vi "MecanumSpeedControlDrive.vi"(0 "RobotDriveDevRef":T1={"DevStatus"={"status"=FALSE, "code"=0, "source"=""}, "Motors[]"=[], "Square Inputs"=FALSE, "Max Output"=1.0}, 1 "Gyro Angle":dbl, 5 "X":dbl, 7 "Array":dbl[](array[numeric]), 9 "Y":dbl, 11 "error in (no error)":errorcluster, 12 "Rotation":dbl) -> (4 "RobotDriveDevRef":T1={"DevStatus"={"status"=FALSE, "code"=0, "source"=""}, "Motors[]"=[], "Square Inputs"=FALSE, "Max Output"=1.0}, 6 "Motor Values":dbl[](array[numeric]), 15 "error out":errorcluster)   [LabVIEW 2014]
doc: "Configures the motors for holonomic driving. Holonomic driving allows you to move the robot in any direction without first rotating or maneuvering the robot.\n\nThis VI requires the robot to have either four omni-directional wheels and four motors mounted at 45 degree angles in the four corners of a square frame or to have four mecanum wheels driven by four motors.\n\nThe control input is intended to be connected directly to the X, Y, and Z axes of a joystick. The Y axis is inverted for you.\n\nThis software is licensed. Open the labview\\readme\\WPI Robotics Library Open Source License.txt file for more information."
uses:
  <vilib>/Rock Robotics/WPI/RobotDrive/WPI_RobotDriveDevRef.ctl
  <vilib>/Rock Robotics/WPI/MotorControl/WPI_MotorControlDeviceRef.ctl
  <vilib>/Rock Robotics/WPI/MotorControl/WPI_MotorControlType.ctl
  <vilib>/Rock Robotics/SystemInterfaces/Typedef/FPGA_TypedefDigitalModule.ctl
  <vilib>/Rock Robotics/SystemInterfaces/DIO/FPGA_DIOPWMChannel.ctl
  <vilib>/Rock Robotics/WPI/PWM/WPI_PWMDeadband.ctl
  <vilib>/Rock Robotics/WPI/CAN/Jaguar/SubVIs/WPI_CANJaguar_ControlMode.ctl
  <vilib>/Rock Robotics/WPI/CAN/TalonSRX/WPI_CANTalonSRX_APIControlMode.ctl
  <vilib>/Rock Robotics/WPI/PWM/WPI_PWMTransform_ConPane.ctl
  <vilib>/Rock Robotics/SystemInterfaces/NetworkCommunication/NetComm_UsageReport_ResourceType.ctl
  <vilib>/Rock Robotics/WPI/RobotDrive/WPI_RobotDriveMotorSelectorEnum.ctl
  <vilib>/Rock Robotics/WPI/RobotDrive/WPI_RobotDriveSafetyCheck.vi
panel:
  out "Front Right":dbl(graph)
  out "Rear Left":dbl(graph)
  out "Rear Right":dbl(graph)
  out "Front Left":dbl(graph)
  out "Right Front":dbl(graph)
  out "Left Front":dbl(graph)
  out "Right Rear":dbl(graph)
  out "Left Rear":dbl(graph)
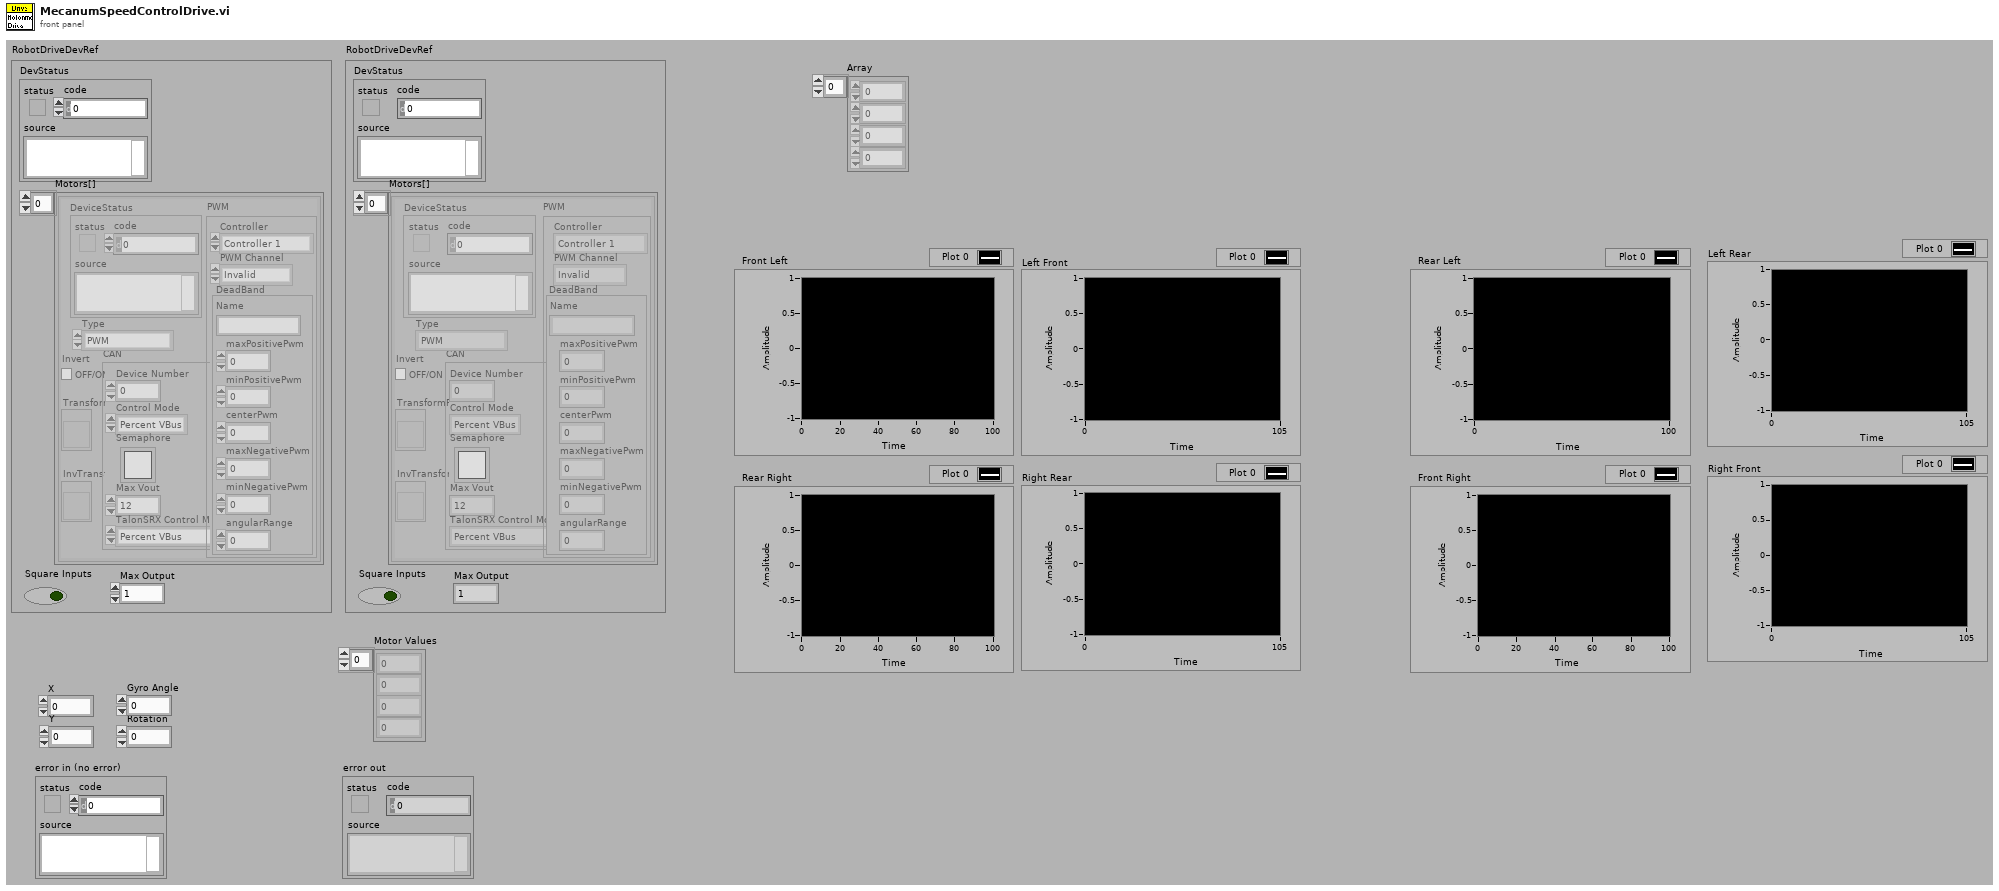
[diagram p1: front panel]
types:
  T1 = typedef "WPI_RobotDriveDevRef.ctl" = cluster{"DevStatus":errorcluster, "Motors[]":T2[], "Square Inputs":bool, "Max Output":dbl}
  T2 = typedef "WPI_MotorControlDeviceRef.ctl" = cluster{"DeviceStatus":errorcluster, "Type":T3, "PWM":cluster{"Controller":T4, "PWM Channel":T5, "DeadBand":T6}, "CAN":cluster{"Device Number":u8, "Control Mode":T7, "Semaphore":T8, "Max Vout":dbl, "TalonSRX Control Mode":T9}, "Invert":bool, "TransformRef":T10, "InvTransformRef":T10}
  T3 = typedef "WPI_MotorControlType.ctl" = enum16{"PWM", "CAN", "CANTalonSRX"}
  T4 = typedef "FPGA_TypedefDigitalModule.ctl" = enum16{"Controller 1"}
  T5 = typedef "FPGA_DIOPWMChannel.ctl" = enum8{"PWM 0", "PWM 1", "PWM 2", "PWM 3", "PWM 4", "PWM 5", "PWM 6", "PWM 7", "PWM 8", "PWM 9", "PWM MXP 0", "PWM MXP 1", "PWM MXP 2", "PWM MXP 3", "PWM MXP 4", "PWM MXP 5", "PWM MXP 6", "PWM MXP 7", "PWM MXP 8", "PWM MXP 9", "Invalid"}
  T6 = typedef "WPI_PWMDeadband.ctl" = cluster{"Name":string, "maxPositivePwm":i32, "minPositivePwm":i32, "centerPwm":i32, "maxNegativePwm":i32, "minNegativePwm":i32, "angularRange":u16}
  T7 = typedef "WPI_CANJaguar_ControlMode.ctl" = enum8{"Percent VBus", "Current", "Speed", "Position", "Voltage"}
  T8 = typedef "Semaphore RefNum" = refnum<k1>
  T9 = typedef "WPI_CANTalonSRX_APIControlMode.ctl" = enum8{"Percent VBus", "Speed", "Position", "Slave", "Unchanged / Invalid"}
  T10 = typedef "WPI_PWMTransform_ConPane.ctl" = refnum<vi>
  T11 = typedef "NetComm_UsageReport_ResourceType.ctl" = enum8{"Controller", "Module", "Language", "CANPlugin", "Accelerometer", "ADXL345", "AnalogChannel", "AnalogTrigger", "AnalogTriggerOutput", "CANJaguar", "Compressor", "Counter", "Dashboard", "DigitalInput", "DigitalOutput", "DriverStationCIO", "DriverStationEIO", "DriverStationLCD", "Encoder", "GearTooth", "Gyro", "I2C", "Framework", "Jaguar", "Joystick", "Kinect", "KinectStick", "PIDController", "Preferences", "PWM", "Relay", "RobotDrive", "SerialPort", "Servo", "Solenoid", "SPI", "Task", "Ultrasonic", "Victor", "Button", "Command", "AxisCamera", "PCVideoServer", "SmartDashboard", "Talon", "HiTechnicColorSensor", "HiTechnicAccel", "HiTechnicCompass", "SRF08", "AnalogOutput", "Victor SP", "Talon SRX", "CAN Talon SRX"}
  T12 = typedef "WPI_RobotDriveMotorSelectorEnum.ctl" = enum16{"Rear Left Motor", "Rear Right Motor", "Front Left Motor", "Front Right Motor"}
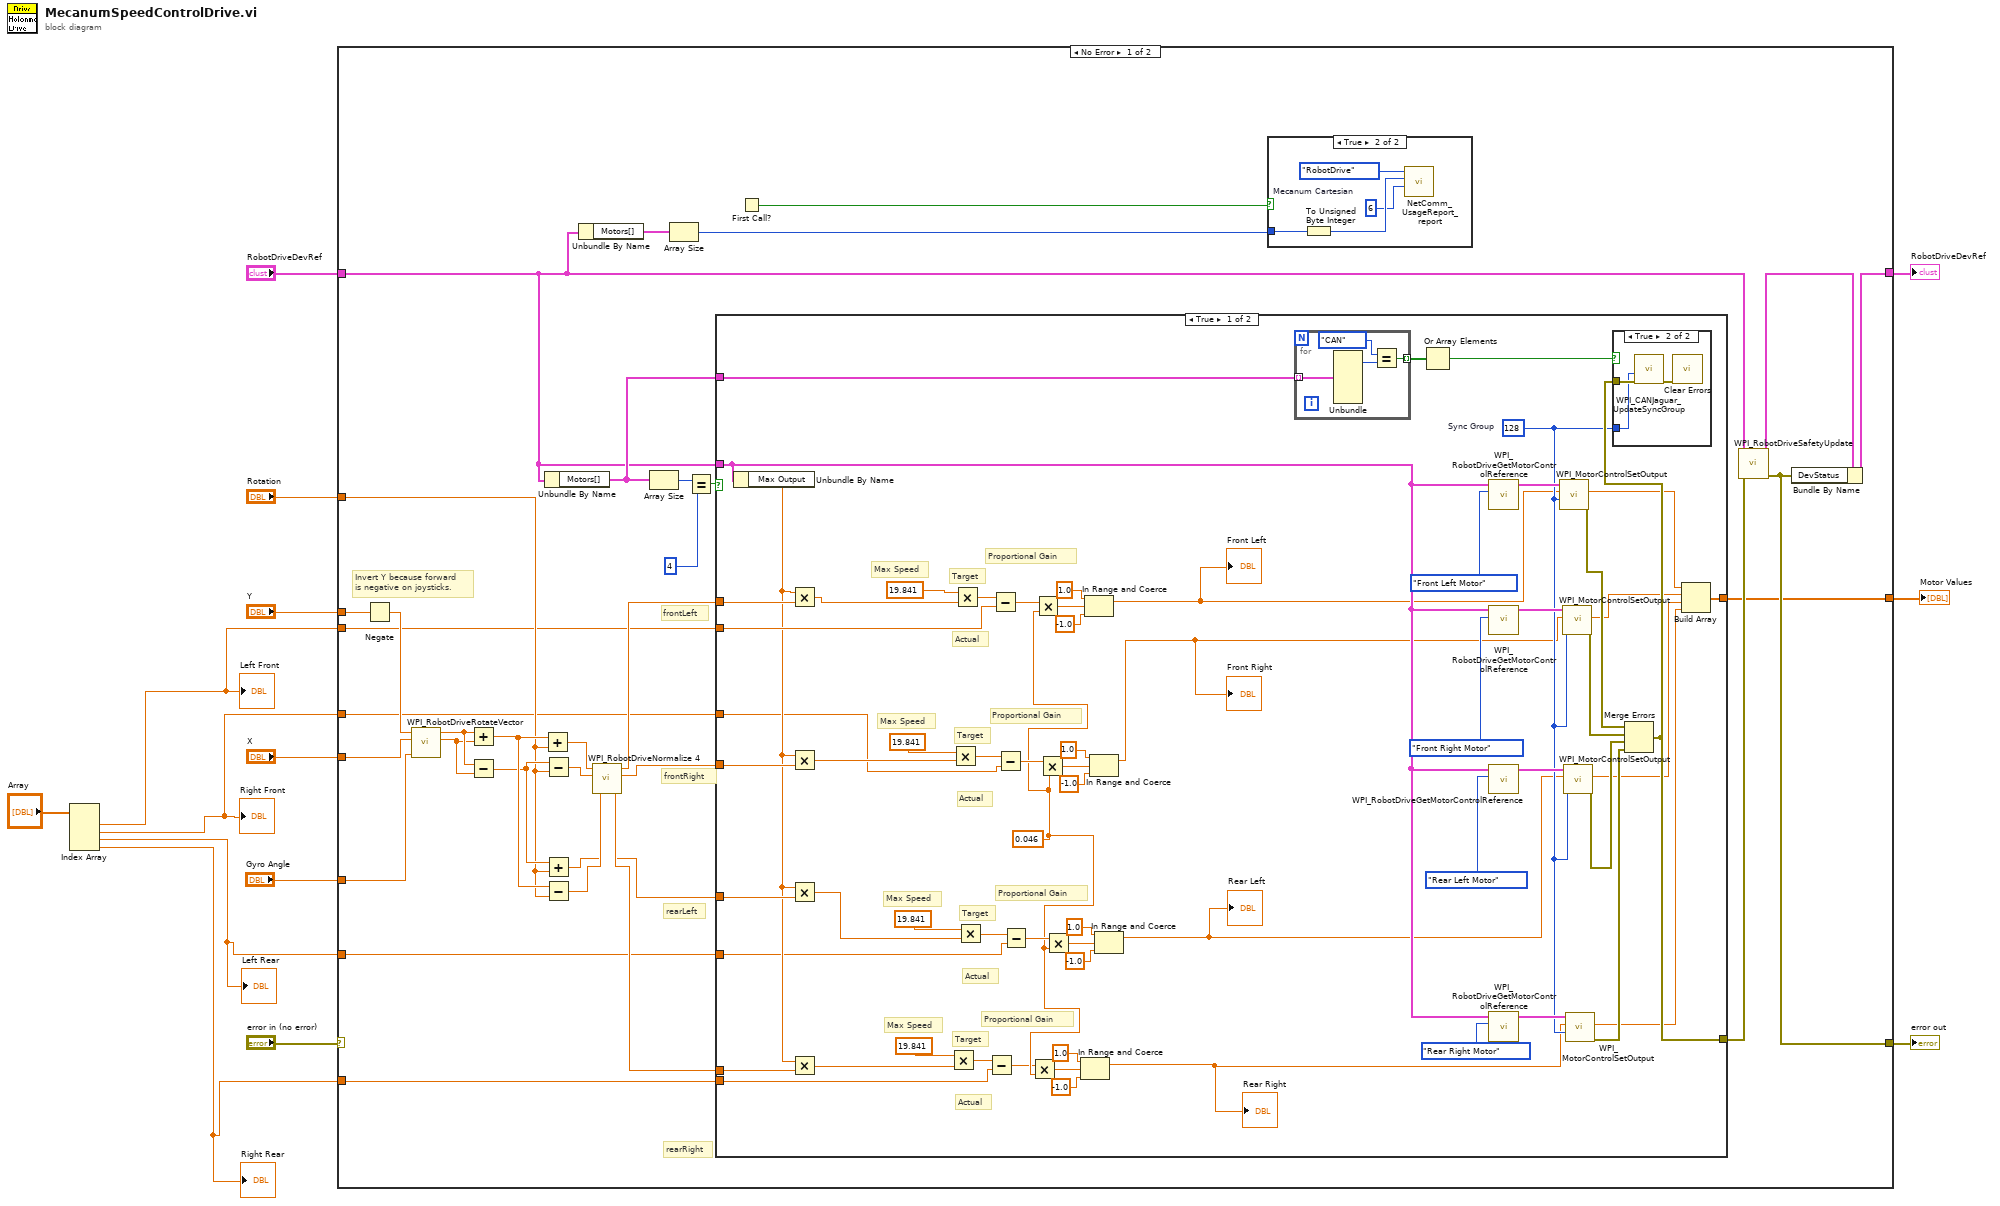
[diagram p0: block diagram]
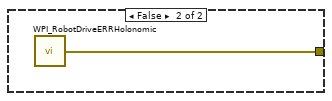
[diagram p4: hidden frame]
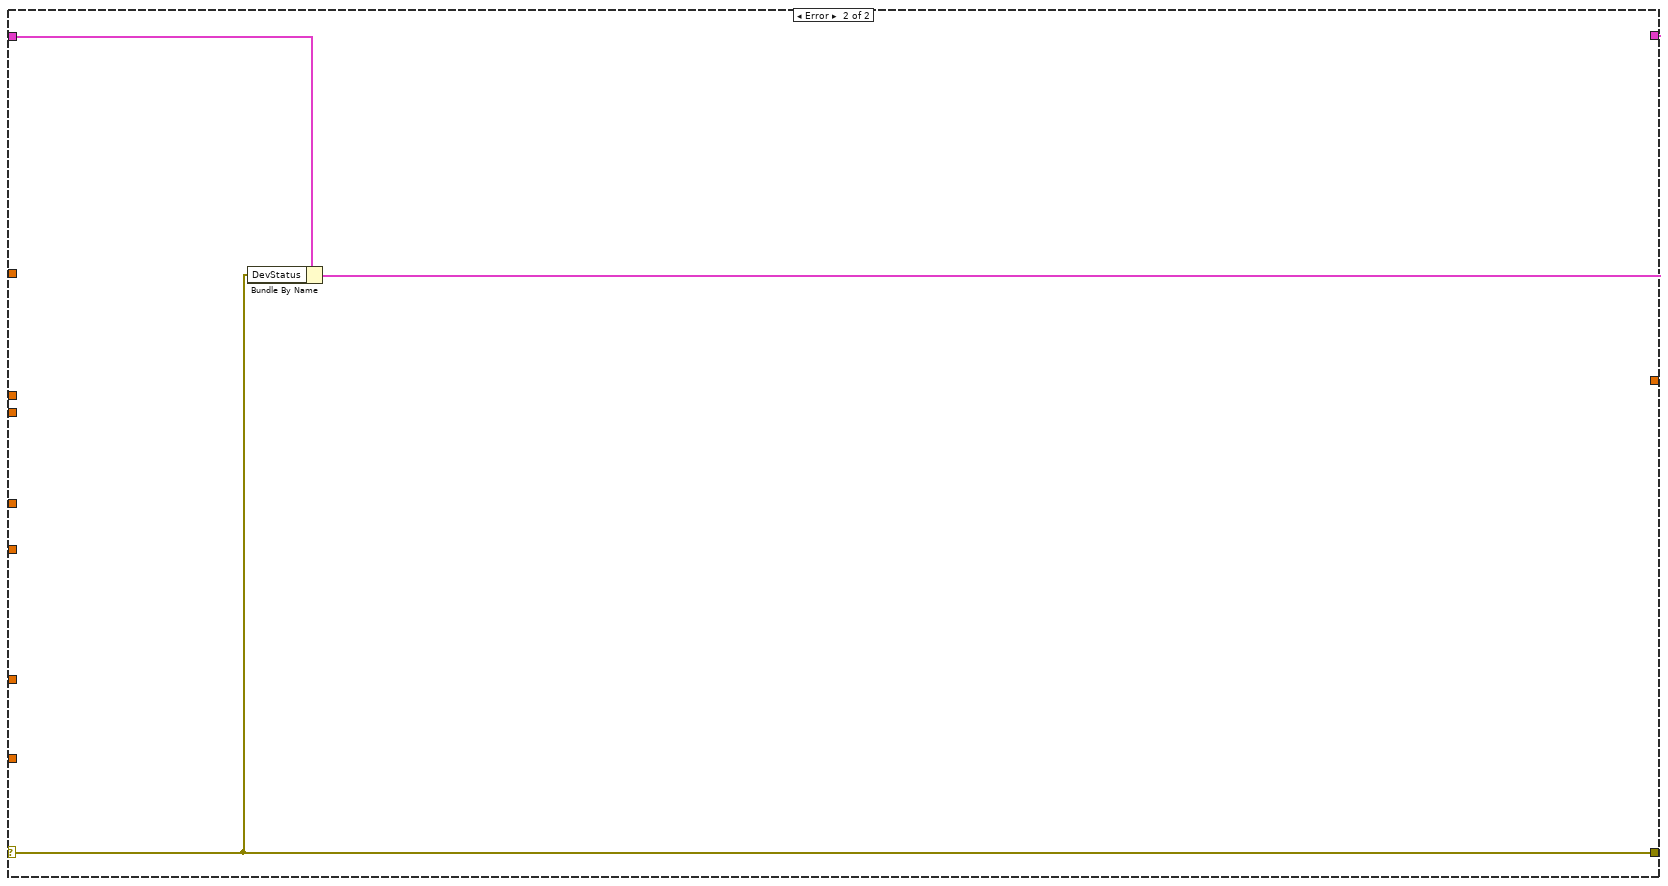
[diagram p5: hidden frame]
diagram:
  n1 = Index Array(array="Array") -> (element #1=w4:dbl, element #2=w3:dbl, element #3=w2:dbl, element #4=w1:dbl)  [unwired: 4 in]
  "Right Front" <- w3
  "Left Front" <- w4
  "Right Rear" <- w1
  "Left Rear" <- w2
  n2 = case shown="No Error" "error in (no error)" {
    selector: "error in (no error)" -> [_ w126]
    tunnel: "Y" -> [w30 _]
    tunnel: "X" -> [w35 _]
    tunnel: "RobotDriveDevRef" -> [w20 w128]
    tunnel: [w45 w127] -> w10
    tunnel: [w25 w126] -> w9
    tunnel: "Rotation" -> [w36 _]
    tunnel: "Gyro Angle" -> [w29 _]
    tunnel: [w19 _] -> w6
    tunnel: w4 -> [w18 _]
    tunnel: w3 -> [w17 _]
    tunnel: w2 -> [w16 _]
    tunnel: w1 -> [w15 _]
    frame No Error {
      # "Invert Y because forward is negative on joysticks."
      # "rearLeft"
      # "frontRight"
      # "rearRight"
      # "frontLeft"
      n3 = Negate(x=w30) -> (-x=w28:dbl)
      n4 = call <vilib>:"WPI_RobotDriveRotateVector.vi"("Angle"=w29, "X"=w35, "Y"=w28) -> ("X'"=w43:dbl, "Y'"=w44:dbl)  [unwired: 7 out]
      n5 = Add(x=w44, y=w43) -> (x+y=w41:dbl)
      n6 = Subtract(x=w44, y=w43) -> (x-y=w39:dbl)
      n7 = Add(x=w41, y=w36) -> (x+y=w37:dbl)
      n8 = Unbundle By Name(w20) -> ("Motors[]"=w24:T2[])
      n9 = Subtract(x=w39, y=w36) -> (x-y=w38:dbl)
      n10 = Add(x=w39, y=w36) -> (x+y=w40:dbl)
      n11 = Subtract(x=w41, y=w36) -> (x-y=w42:dbl)
      n12 = Unbundle By Name(w20) -> ("Motors[]"=w22:T2[])
      n13 = call <vilib>:"WPI_RobotDriveNormalize 4.vi"("D"=w42, "C"=w40, "B"=w38, "A"=w37) -> ("D'"=w32:dbl, "C'"=w31:dbl, "B'"=w33:dbl, "A'"=w34:dbl)
      n14 = Array Size(array=w24) -> (size(s)=w48:i32)
      n15 = Array Size(array=w22) -> (size(s)=w21:i32)
      n16 = Equal?(x=w48, y=4) -> (x = y?=w46:bool)
      n17 = case shown="True" w46 {
        tunnel: w34 -> [w117 _]
        tunnel: w33 -> [w116 _]
        tunnel: w20 -> [w105 _]
        tunnel: [w97 w125] -> w27
        tunnel: w31 -> [w111 _]
        tunnel: w32 -> [w110 _]
        tunnel: w24 -> [w98 _]
        tunnel: [w94 _] -> w19
        tunnel: w18 -> [w86 _]
        tunnel: w17 -> [w67 _]
        tunnel: w16 -> [w66 _]
        tunnel: w15 -> [w65 _]
        frame True {
          w64 = 0.046
          w96 = u8 128  # Sync Group
          # "Max Speed"
          # "Proportional Gain"
          # "Actual"
          # "Target"
          # "Max Speed"
          # "Proportional Gain"
          # "Actual"
          # "Target"
          # "Max Speed"
          # "Proportional Gain"
          # "Actual"
          # "Target"
          # "Max Speed"
          # "Proportional Gain"
          # "Actual"
          # "Target"
          n18 = Unbundle By Name(w105) -> ("Max Output"=w85:dbl)
          n19 = Multiply(x=w85, y=w117) -> (x*y=w83:dbl)
          n20 = Multiply(x=w85, y=w116) -> (x*y=w69:dbl)
          n21 = Multiply(x=w85, y=w111) -> (x*y=w68:dbl)
          n22 = Multiply(x=w85, y=w110) -> (x*y=w54:dbl)
          n23 = Multiply(x=19.841, y=w54) -> (x*y=w60:dbl)
          n24 = Multiply(x=19.841, y=w69) -> (x*y=w76:dbl)
          n25 = Multiply(x=19.841, y=w83) -> (x*y=w84:dbl)
          n26 = Multiply(x=19.841, y=w68) -> (x*y=w75:dbl)
          n27 = Subtract(x=w60, y=w65) -> (x-y=w59:dbl)
          n28 = Subtract(x=w84, y=w86) -> (x-y=w90:dbl)
          n29 = Subtract(x=w76, y=w67) -> (x-y=w77:dbl)
          n30 = Subtract(x=w75, y=w66) -> (x-y=w74:dbl)
          n31 = Multiply(x=w59, y=w64) -> (x*y=w58:dbl)
          n32 = Multiply(x=w90, y=w64) -> (x*y=w89:dbl)
          n33 = Multiply(x=w77, y=w64) -> (x*y=w78:dbl)
          n34 = Multiply(x=w74, y=w64) -> (x*y=w73:dbl)
          n35 = In Range and Coerce(upper limit=1.0, x=w58, lower limit=-1.0) -> (coerced(x)=w53:dbl)  [unwired: 1 out]
          "Rear Right" <- w53
          n36 = In Range and Coerce(upper limit=1.0, x=w89, lower limit=-1.0) -> (coerced(x)=w61:dbl)  [unwired: 1 out]
          "Front Left" <- w61
          n37 = In Range and Coerce(upper limit=1.0, x=w78, lower limit=-1.0) -> (coerced(x)=w62:dbl)  [unwired: 1 out]
          "Front Right" <- w62
          n38 = In Range and Coerce(upper limit=1.0, x=w73, lower limit=-1.0) -> (coerced(x)=w63:dbl)  [unwired: 1 out]
          "Rear Left" <- w63
          n39 = for {
            tunnel: w98 -> [w121] mode=indexing
            tunnel: [w118] -> w99 mode=indexing
            n40 = Unbundle(w121) -> ("Type"=w120:T3)  [unwired: 6 out]
            n41 = Equal?(x=enum16{"PWM", "CAN"}."CAN" ("Type"), y=w120) -> (x = y?=w118:bool)
          }
          n42 = Or Array Elements(Boolean array=w99) -> (logical OR=w100:bool)
          n43 = call <vilib>:"WPI_RobotDriveGetMotorControlReference.vi"("MotorIndex"=WPI_RobotDriveMotorSelectorEnum."Front Left Motor", "RobotDriveDevRef"=w105) -> ("MotorControlDeviceRef"=w115:T2)  [unwired: 9 out]
          n44 = call <vilib>:"WPI_RobotDriveGetMotorControlReference.vi"("MotorIndex"=WPI_RobotDriveMotorSelectorEnum."Front Right Motor", "RobotDriveDevRef"=w105) -> ("MotorControlDeviceRef"=w113:T2)  [unwired: 9 out]
          n45 = call <vilib>:"WPI_RobotDriveGetMotorControlReference.vi"("MotorIndex"=WPI_RobotDriveMotorSelectorEnum."Rear Left Motor", "RobotDriveDevRef"=w105) -> ("MotorControlDeviceRef"=w114:T2)  [unwired: 9 out]
          n46 = call <vilib>:"WPI_RobotDriveGetMotorControlReference.vi"("MotorIndex"=WPI_RobotDriveMotorSelectorEnum."Rear Right Motor", "RobotDriveDevRef"=w105) -> ("MotorControlDeviceRef"=w112:T2)  [unwired: 9 out]
          n47 = call <vilib>:"WPI_MotorControlSetOutput.vi"("Sync Group / Parameter Slot"=w96, "Output"=w61, "MotorControlDevRef"=w115) -> ("error out"=w101:errorcluster, "Motor Output"=w95:dbl)  [unwired: 2 in, 5 out]
          n48 = call <vilib>:"WPI_MotorControlSetOutput.vi"("Sync Group / Parameter Slot"=w96, "Output"=w62, "MotorControlDevRef"=w113) -> ("error out"=w102:errorcluster, "Motor Output"=w93:dbl)  [unwired: 2 in, 5 out]
          n49 = call <vilib>:"WPI_MotorControlSetOutput.vi"("Sync Group / Parameter Slot"=w96, "Output"=w63, "MotorControlDevRef"=w114) -> ("error out"=w103:errorcluster, "Motor Output"=w92:dbl)  [unwired: 2 in, 5 out]
          n50 = call <vilib>:"WPI_MotorControlSetOutput.vi"("Sync Group / Parameter Slot"=w96, "Output"=w53, "MotorControlDevRef"=w112) -> ("error out"=w104:errorcluster, "Motor Output"=w91:dbl)  [unwired: 2 in, 5 out]
          n51 = Merge Errors(w101, w102, w103, w104) -> (w97:errorcluster)
          n52 = case shown="True" w100 {
            tunnel: w97 -> [_ w123]
            tunnel: w96 -> [_ w122]
            frame False {
            }
            frame True {
              n53 = call <vilib>:"WPI_CANJaguar_UpdateSyncGroup.vi"("error in (no error)"=w123, "Sync Group"=w122) -> ("error out"=w124:errorcluster)  [unwired: 9 out]
              n54 = call <vilib>:"Clear Errors.vi"("error in (no error)"=w124) -> ()  [unwired: 1 in, 6 out]
            }
          }
          n55 = Build Array(w95, w93, w92, w91) -> (w94:dbl[])
        }
        frame False {
          n56 = call <vilib>:"WPI_RobotDriveERRHolonomic.vi"() -> ("error out"=w125:errorcluster)
        }
      }
      n57 = First Call?() -> (First Call?: T/F=w23:bool)
      n58 = case shown="True" w23 {
        tunnel: w21 -> [_ w51]
        frame False {
        }
        frame True {
          w49 = u8 6  # Mecanum Cartesian
          n59 = To Unsigned Byte Integer(number=w51) -> (unsigned 8bit integer=w50:u8)
          n60 = call <vilib>:"NetComm_UsageReport_report.vi"("Context"=w49, "Instance Number"=w50, "Resource Type"=NetComm_UsageReport_ResourceType."RobotDrive") -> ()  [unwired: 9 in]
        }
      }
      n61 = call <vilib>:"WPI_RobotDriveSafetyUpdate.vi"("error in (no error)"=w27, "RobotDriveDevRef"=w20) -> ("error out"=w25:errorcluster, "RobotDriveDevRef"=w26:T1)  [unwired: 8 out]
      n62 = Bundle By Name(cluster=w26, "DevStatus"=w25) -> (w45:T1)
    }
    frame Error {
      n63 = Bundle By Name(cluster=w128, "DevStatus"=w126) -> (w127:T1)
    }
  }
  "error out" <- w9
  "RobotDriveDevRef" <- w10
  "Motor Values" <- w6
